vi "IVA_Actividad_01.vi"() -> ()   [LabVIEW 2025]
uses:
  <vilib>/Instr/_visa.llb/VISA Configure Serial Port (Instr).vi
panel:
  out "Contador":dbl(knob) scale=-100.0..100.0
  out "Termómetro":dbl(slide) scale=10.0..50.0
  out "contador":string
  out "temperatura":string
  in  "stop":bool
  in  "VISA resource name":refnum<visa-resource-name>
  out "read buffer":string
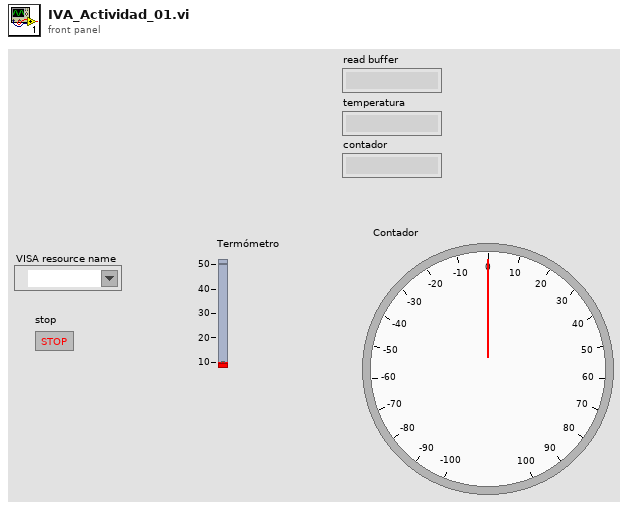
[diagram p1: front panel]
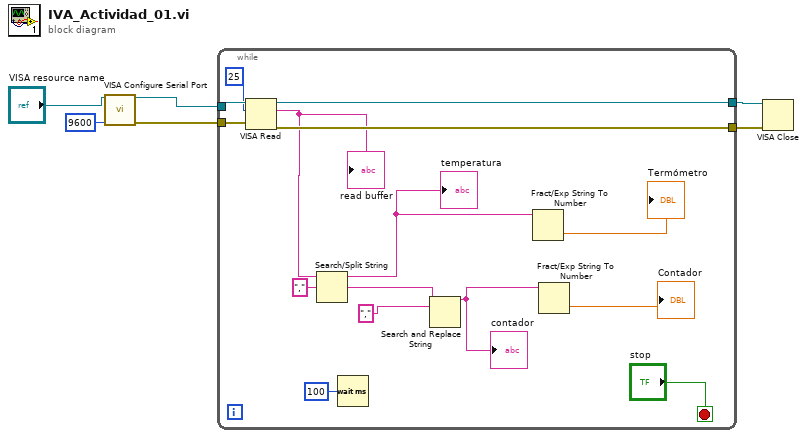
[diagram p0: block diagram]
diagram:
  n1 = call-poly "VISA Configure Serial Port"("VISA resource name"="VISA resource name", "baud rate (9600)"=u32 9600) -> ("VISA resource name out"=w5:refnum<visa-resource-name>, "error out"=w3:errorcluster)  [unwired: 12 in]
  n2 = while {
    tunnel: w5 -> [w20]
    tunnel: [w18] -> w4
    tunnel: w3 -> [w17]
    tunnel: [w16] -> w2
    stop <- "stop" stop-if-true
    n3 = VISA Read(VISA resource name=w20, byte count=u32 25, error in (no error)=w17) -> (VISA resource name out=w18:refnum<visa-resource-name>, read buffer=w13:string, error out=w16:errorcluster)  [unwired: 1 out]
    "read buffer" <- w13
    n4 = Search/Split String(string=w13, search string/char (-)=",") -> (substring before match=w12:string, match + rest of string=w8:string)  [unwired: 1 in, 1 out]
    "temperatura" <- w12
    n5 = Wait (ms)(milliseconds to wait=u32 100) -> ()  [unwired: 1 out]
    n6 = Search and Replace String(input string=w8, search string=",") -> (result string=w9:string)  [unwired: 6 in, 3 out]
    "contador" <- w9
    n7 = Fract/Exp String To Number(string=w12) -> (number=→"Termómetro":dbl)  [unwired: 3 in, 1 out]
    n8 = Fract/Exp String To Number(string=w9) -> (number=→"Contador":dbl)  [unwired: 3 in, 1 out]
  }
  n9 = VISA Close(VISA resource name=w4, error in (no error)=w2) -> ()  [unwired: 1 out]
